vi "Test Cluster with Two Elements.vi"(11 "Test Case In":refnum<class "Describe Variant Test.lvclass">) -> (0 "error out":errorcluster, 3 "Test Case Out":refnum<class "Describe Variant Test.lvclass">)   [LabVIEW 2020, in "Describe Variant Test.lvclass"]
uses:
  Describe Variant Test.lvclass
  Describe Variant Test.lvclass/Describe Variant Test.ctl
  source/Framework/Utilities/Utilities.lvlib
  98c118be-9cde-43f8-b72f-2f839d52d121.vi
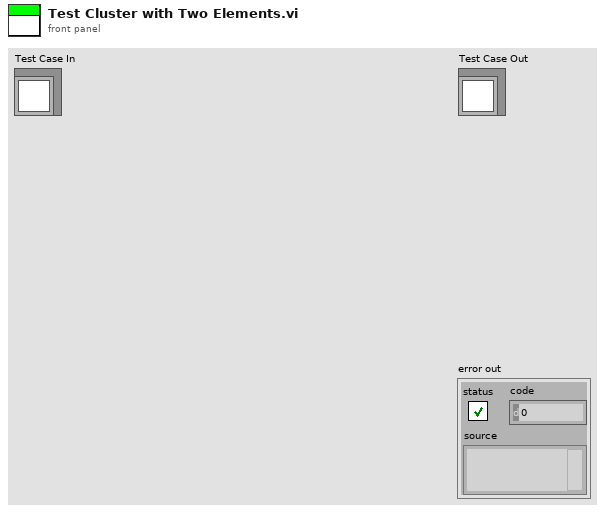
[diagram p1: front panel]
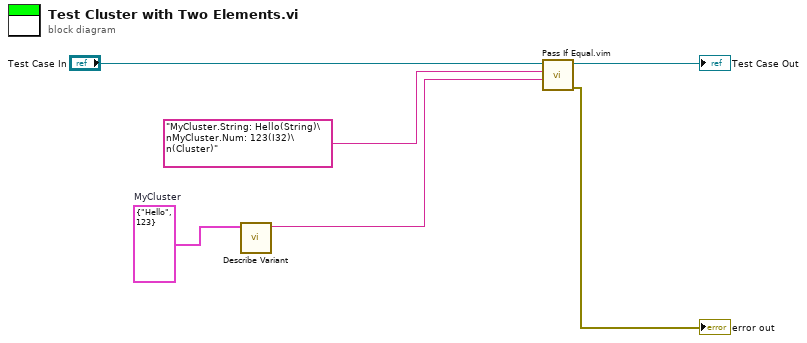
[diagram p0: block diagram]
diagram:
  w1 = cluster{"String":string, "Num":i32} {"String"="Hello", "Num"=123}  # MyCluster
  n1 = call "Describe Variant.vi"("Variant"=w1) -> ("Variant Description"=w2:string)  [unwired: 8 in, 2 out]
  n2 = call "Pass If Equal.vim"("Actual"=w2, "Expected"="MyCluster.String: Hello(String)\nMyCluster.Num: 123(I32)\n(Cluster)", "LUnit Test Case In"="Test Case In") -> ("error out"=→"error out":errorcluster, "LUnit Test Case Out"=→"Test Case Out":refnum<class "Describe Variant Test.lvclass">)  [unwired: 7 in]
